vi "Write_to_file.vi"(1 "Data to be logged":string, 2 "File header if log file is empty":string, 3 "file path (use dialog)":path) -> ()   [LabVIEW 2023]
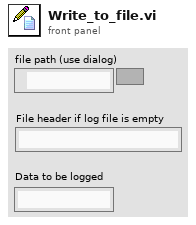
[diagram p1: front panel]
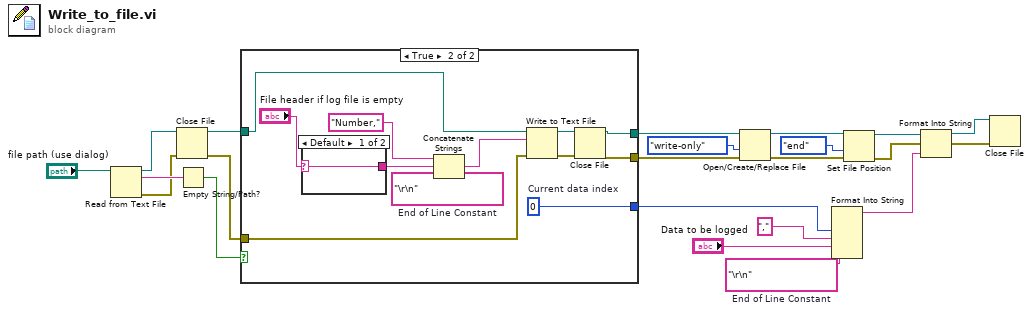
[diagram p0: block diagram]
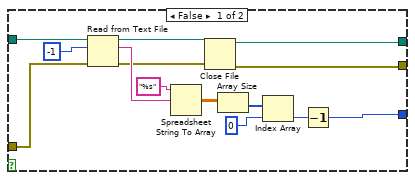
[diagram p2: hidden frame]
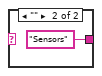
[diagram p3: hidden frame]
diagram:
  w2 = "\r\n"  # End of Line Constant
  n1 = Read from Text File(file (use dialog)="file path (use dialog)") -> (refnum out=w14:refnum<file>, text=w16:string, error out=w12:errorcluster)  [unwired: 3 in, 1 out]
  n2 = Close File(refnum=w14, error in=w12) -> (path=w13:path, error out=w11:errorcluster)
  n3 = Empty String/Path?(string/path=w16) -> (empty?=w17:bool)
  n4 = case shown="True" w17 {
    tunnel: w13 -> [w36 w38]
    tunnel: w11 -> [w35 w48]
    tunnel: [w23 w44] -> w10
    tunnel: [w24 w43] -> w9
    tunnel: [w31 w42] -> w5
    frame False {
      n5 = Read from Text File(file (use dialog)=w36, count=-1, error in=w35) -> (refnum out=w26:refnum<file>, text=w33:string, error out=w25:errorcluster)  [unwired: 1 in, 1 out]
      n6 = Spreadsheet String To Array(format string="%s", spreadsheet string=w33) -> (array=w32:dbl[][])  [unwired: 2 in]
      n7 = Close File(refnum=w26, error in=w25) -> (path=w23:path, error out=w24:errorcluster)
      n8 = Array Size(array=w32) -> (size(s)=w28:i32[])
      n9 = Index Array "Index Array"(array=w28, index=0) -> (element=w29:i32)
      n10 = Decrement(x=w29) -> (x-1=w31:i32)
    }
    frame True {
      w40 = "\r\n"  # End of Line Constant
      w42 = 0  # Current data index
      n11 = case shown="Default" "File header if log file is empty" {
        selector: "File header if log file is empty" -> [w49 _]
        tunnel: [w49 "Sensors"] -> w37
        frame Default {
        }
        frame "" {
        }
      }
      n12 = Concatenate Strings("Number,", w37, w40) -> (w47:string)
      n13 = Write to Text File(file (use dialog)=w38, text=w47, error in=w48) -> (refnum out=w46:refnum<file>, error out=w45:errorcluster)  [unwired: 1 in, 1 out]
      n14 = Close File(refnum=w46, error in=w45) -> (path=w44:path, error out=w43:errorcluster)
    }
  }
  n15 = Open/Create/Replace File(file path (use dialog)=w10, error in=w9, access (0:read/write)=enum16{"read/write", "read-only", "write-only"}."write-only") -> (refnum out=w22:refnum<file>, error out=w8:errorcluster)  [unwired: 3 in, 1 out]
  n16 = Format Into String(w5, "," ("text"), "Data to be logged", w2) -> (resulting string=w4:string)  [unwired: 3 in, 1 out]
  n17 = Set File Position(refnum=w22, from (0:start)=enum16{"start", "end", "current"}."end", error in=w8) -> (refnum out=w21:refnum<file>, error out=w7:errorcluster)  [unwired: 1 in]
  n18 = Format Into String(initial string=w21, error in=w7, w4) -> (resulting string=w20:refnum<file>, error out=w6:errorcluster)  [unwired: 1 in]
  n19 = Close File(refnum=w20, error in=w6) -> ()  [unwired: 2 out]
